vi "Find DO Tags.vi"(8 "error in (no error)":errorcluster, 11 "DAQ State in":T1) -> (0 "error out":errorcluster, 2 "Task D-O Channels":string[][](array[string]), 3 "DAQ State out":T1)   [LabVIEW 2018, in "DAQ.lvlib"]
uses:
  DAQ/DAQ.lvlib
  Hardware Configuration.ctl
  Task Cluster.ctl
  <resource>/objmgr/daqmx.rc
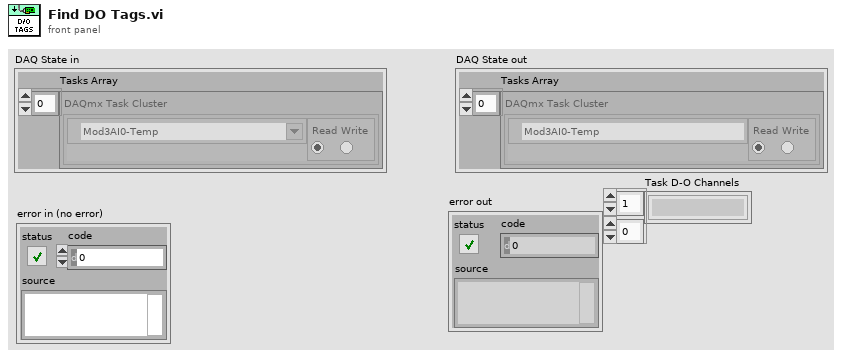
[diagram p1: front panel]
types:
  T1 = typedef "DAQ.lvlib/Hardware Configuration.ctl" = cluster{"Tasks Array":T2[]}
  T2 = typedef "Task Cluster.ctl" = cluster{"DAQmx Task":refnum<k21>, "Read-Write Radio":enum32{"Read", "Write"}}
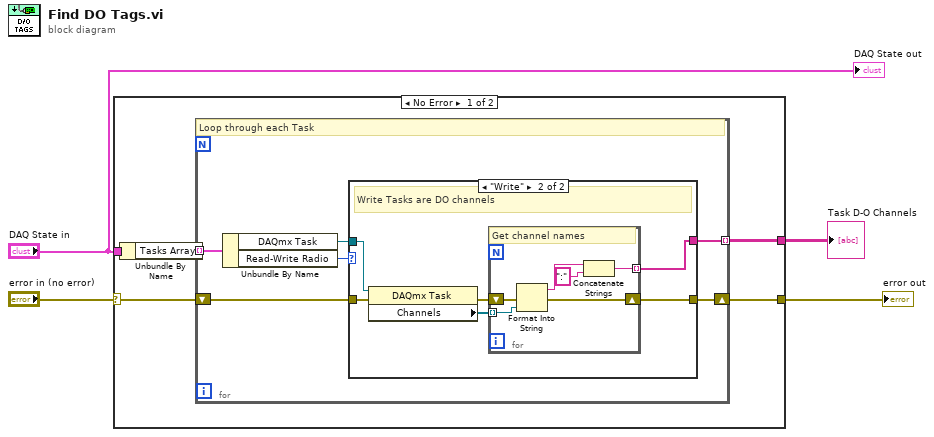
[diagram p0: block diagram]
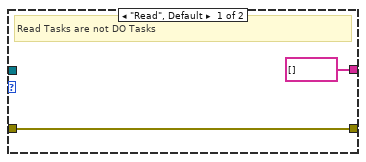
[diagram p2: hidden frame]
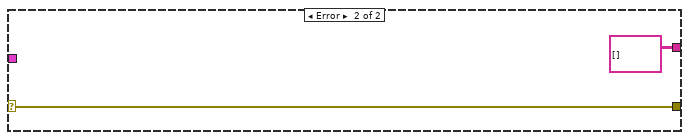
[diagram p3: hidden frame]
diagram:
  n1 = case shown="No Error" "error in (no error)" {
    selector: "error in (no error)" -> [w6 w31]
    tunnel: "DAQ State in" -> [w8 _]
    tunnel: [w7 w31] -> w2
    tunnel: [w5 string[][] []] -> w1
    frame No Error {
      n2 = Unbundle By Name(w8) -> ("Tasks Array"=w9:T2[])
      n3 = for {
        tunnel: w9 -> [w15] mode=indexing
        shift-right: [w12] -> w7
        shift-left: w6 -> [w10]
        tunnel: [w13] -> w5 mode=indexing
        # "Loop through each Task"
        n4 = Unbundle By Name(w15) -> ("DAQmx Task"=w11:refnum<k21>, "Read-Write Radio"=w14:enum32{"Read", "Write"})
        n5 = case shown="\"Write\"" w14 {
          tunnel: [string[] [] w18] -> w13
          tunnel: [w17 w23] -> w12
          tunnel: w11 -> [_ w22]
          tunnel: w10 -> [w17 w21]
          frame "Read", Default {
            # "Read Tasks are not DO Tasks"
          }
          frame "Write" {
            # "Write Tasks are DO channels"
            n6 = property class="DAQmx Task"(reference=w22, error in=w21) -> (error out=w20:errorcluster, "Channels"=w19:refnum<k21>[])  [unwired: 1 out]
            n7 = for {
              tunnel: w19 -> [w29] mode=indexing
              shift-right: [w27] -> w23
              shift-left: w20 -> [w28]
              tunnel: [w24] -> w18 mode=indexing
              # "Get channel names"
              n8 = Format Into String(error in=w28, w29) -> (resulting string=w26:string, error out=w27:errorcluster)  [unwired: 2 in]
              n9 = Concatenate Strings(w26, ":" ("string")) -> (w24:string)
            }
          }
        }
      }
    }
    frame Error {
    }
  }
  "error out" <- w2
  "Task D-O Channels" <- w1
  "DAQ State out" <- "DAQ State in"
